vi "Send Message.vi"(8 "error in (no error)":errorcluster, 10 "Message":refnum<class "Message.lvclass">, 11 "Endpoint in":refnum<class "Endpoint.lvclass">) -> (0 "error out":errorcluster, 3 "Endpoint out":refnum<class "Endpoint.lvclass">)   [LabVIEW 2020, in "Stream-Simple-Msg.lvlib" / "Endpoint.lvclass"]
uses:
  Endpoint.lvclass
  Message/Message.lvclass
  Endpoint.lvclass/Endpoint.ctl
  lv-stream/stream/Stream/Stream.lvclass
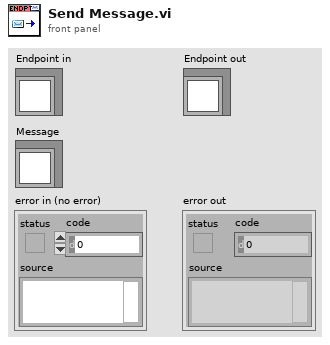
[diagram p1: front panel]
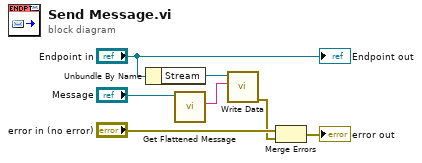
[diagram p0: block diagram]
diagram:
  n1 = Unbundle By Name("Endpoint in") -> ("Stream"=w4:refnum<class "Stream.lvclass">)
  n2 = call "Get Flattened Message.vi"("Message in"="Message") -> ("Flattened Message"=w3:string)  [unwired: 8 in, 2 out]
  n3 = call-dynamic "Write Data.vi"("Data"=w3, "Stream in"=w4) -> ("error out"=w1:errorcluster)  [unwired: 8 in, 1 out]
  n4 = Merge Errors("error in (no error)", w1) -> (→"error out":errorcluster)
  "Endpoint out" <- "Endpoint in"
